vi "Set UIPosition.vi"(8 "error in":errorcluster, 9 "VI Ref":refnum<vi>, 11 "Sequence Context In":refnum<k7>) -> (0 "error out":errorcluster, 1 "reference out":refnum<vi>, 3 "Sequence Context Out":refnum<k7>)   [LabVIEW 2019, in "OPC UA.lvlib" / "TestExec.lvclass"]
uses:
  TestExec.lvclass
  <vilib>/addons/TestStand/_TSUtility.llb/TestStand - Get Property Value (Number).vi
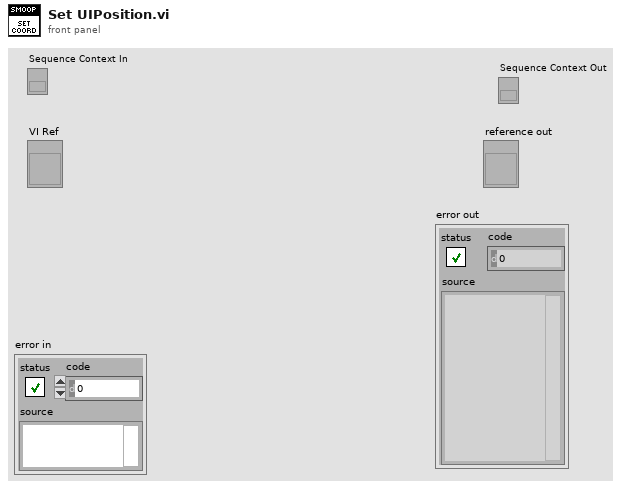
[diagram p1: front panel]
types:
  T1 = typedef "LVRectTypeDef.ctl" = cluster{"Left":i16, "Top":i16, "Right":i16, "Bottom":i16}
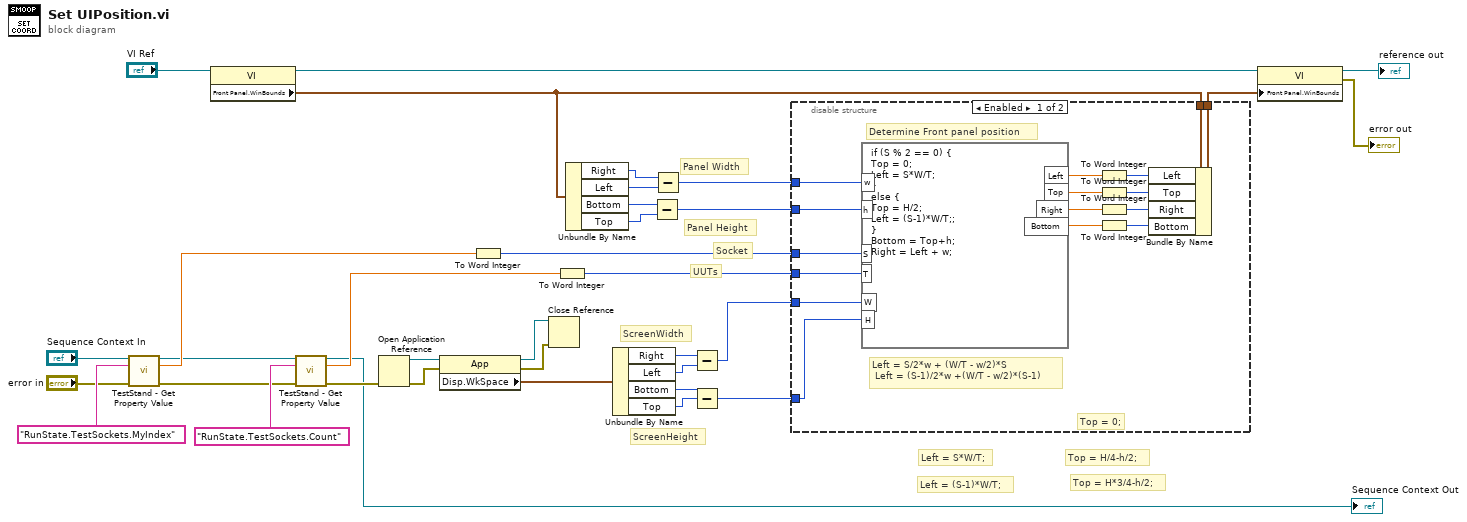
[diagram p0: block diagram]
diagram:
  # "Top = H*3/4-h/2;"
  # "Top = H/4-h/2;"
  # "Left = (S-1)*W/T;"
  # "Left = S*W/T;"
  # "UUTs"
  # "Socket"
  # "Panel Height"
  # "Panel Width"
  # "ScreenHeight"
  # "ScreenWidth"
  n1 = call-poly <vilib>:"TestStand - Get Property Value.vi"("Sequence Context In"="Sequence Context In", "Lookup String"="RunState.TestSockets.MyIndex", "error in (no error)"="error in") -> ("Sequence Context Out"=w6:refnum<k7>, "Value"=w25:dbl, "error out"=w5:errorcluster)  [unwired: 10 in]
  n2 = property class="VI"(reference="VI Ref") -> (reference out=w29:refnum<vi>, "Front Panel.WinBounds"=w35:T1)  [unwired: 1 in, 1 out]
  n3 = call-poly <vilib>:"TestStand - Get Property Value.vi"("Sequence Context In"=w6, "Lookup String"="RunState.TestSockets.Count", "error in (no error)"=w5) -> ("Sequence Context Out"=→"Sequence Context Out":refnum<k7>, "Value"=w24:dbl, "error out"=w21:errorcluster)  [unwired: 10 in]
  n4 = Open Application Reference(8:w21) -> (0:w23:errorcluster, 3:w22:refnum<vi>)  [unwired: 3 in]
  n5 = property class="App"(reference=w22, error in=w23) -> (reference out=w13:refnum<vi>, error out=w12:errorcluster, "Disp.WkSpace"=w20:T1)
  n6 = To Word Integer(number=w25) -> (16bit integer=w3:i16)
  n7 = Close Reference(reference=w13, error in (no error)=w12) -> ()  [unwired: 1 out]
  n8 = To Word Integer(number=w24) -> (16bit integer=w4:i16)
  n9 = Unbundle By Name(w35) -> ("Right"=w34:i16, "Left"=w33:i16, "Bottom"=w32:i16, "Top"=w31:i16)
  n10 = Unbundle By Name(w20) -> ("Right"=w19:i16, "Left"=w18:i16, "Bottom"=w17:i16, "Top"=w16:i16)
  n11 = Subtract(x=w32, y=w31) -> (x-y=w27:i16)
  n12 = Subtract(x=w34, y=w33) -> (x-y=w28:i16)
  n13 = Subtract(x=w19, y=w18) -> (x-y=w15:i16)
  n14 = Subtract(x=w17, y=w16) -> (x-y=w14:i16)
  n15 = disable-structure shown="Enabled" {
    disable-tunnel: w35 -> [w51 w52]
    disable-tunnel: w28 -> [w50 _]
    disable-tunnel: w27 -> [w49 _]
    disable-tunnel: [w41 w52] -> w26
    disable-tunnel: w3 -> [w39 _]
    disable-tunnel: w4 -> [w38 _]
    disable-tunnel: w15 -> [w37 _]
    disable-tunnel: w14 -> [w36 _]
    frame Enabled {
      # "Top = 0;"
      # "Left = S/2*w + (W/T - w/2)*S\n Left = (S-1)/2*w +(W/T - w/2)*(S-1)"
      # "Determine Front panel position"
      n16 = formula code="if (S % 2 == 0) {\nTop = 0;\nLeft = S*W/T;\n}\nelse {\nTop = H/2;\nLeft = (S-1)*W/T;;\n}\nBottom = Top+h;\nRight = Left + w;"("S"=w39, "T"=w38, "W"=w37, "H"=w36, "w"=w50, "h"=w49) -> ("Left"=w45:dbl, "Top"=w48:dbl, "Right"=w47:dbl, "Bottom"=w46:dbl)
      n17 = To Word Integer(number=w45) -> (16bit integer=w40:i16)
      n18 = To Word Integer(number=w48) -> (16bit integer=w44:i16)
      n19 = To Word Integer(number=w47) -> (16bit integer=w43:i16)
      n20 = To Word Integer(number=w46) -> (16bit integer=w42:i16)
      n21 = Bundle By Name(cluster=w51, "Left"=w40, "Top"=w44, "Right"=w43, "Bottom"=w42) -> (w41:T1)
    }
    frame Disabled {
    }
  }
  n22 = property on="Property Node" class="VI"(reference=w29, "Front Panel.WinBounds"=w26) -> (reference out=→"reference out":refnum<vi>, error out=→"error out":errorcluster)  [unwired: 1 in]
